vi "ni5660 Read FFT Spectrum.vi"(0 "receiver info in":T2, 9 "correction factor":T1[](array[typedef]) {"spectrum correction"."correction factors" format="%.2f"; "spectrum correction"."df" format="%.2f"; "spectrum correction"."f0" format="%.2f"}, 11 "error in (no error)":errorcluster) -> (4 "receiver info out":T2, 6 "FFT spectrum (Vrms)":cluster{"f0":dbl, "df":dbl, "spectrum":cdb[]} {"spectrum" format="%.2f"; "df" format="%.2f"; "f0" format="%.2f"}, 8 "spectral info out":T3={"spectrum type"=enum."Power [Magnitude^2]", "linear/dB"=enum."linear", "window"=0, "window size"=1024, "FFT size"=1024} {"window" items=["None ", "Hanning", "Hamming", "Blackman-Harris", "Exact Blackman", "Blackman", "Flat Top", "4 Term B-Harris ", "7 Term B-Harris", "Low Sidelobe"]}, 15 "error out":errorcluster)   [LabVIEW 2011]
doc: "This VI computes the FFT spectrum that corresponds to the spectral settings specified in the ni5660 Configure for Spectrum VI. The VI returns a cluster that contains the FFT spectrum in Vrms, starting at frequency <B>f0</B> and frequency interval <B>df</B>. Wire the <B>FFT spectrum</B> output to averaging and/or measurement VIs in the Spectral Measurements Toolkit."
uses:
  <vilib>/measure/masml.llb/ma_sml_Spectral Info.ctl
  <vilib>/addons/Modulation/niScope/controls/mod_Modulation Settings.ctl
  <vilib>/addons/Spectral Measurements Toolset/LVSupport/SMT niScope Utilities/smt_correction.ctl
  <vilib>/addons/Spectral Measurements Toolset/LVSupport/SMT niScope Utilities/smt_Apply Correction(FFT).vi
  <vilib>/addons/Spectral Measurements Toolset/SMT Zoom FFT for niScope.vi
  <vilib>/measure/NI_MAPro.lvlib
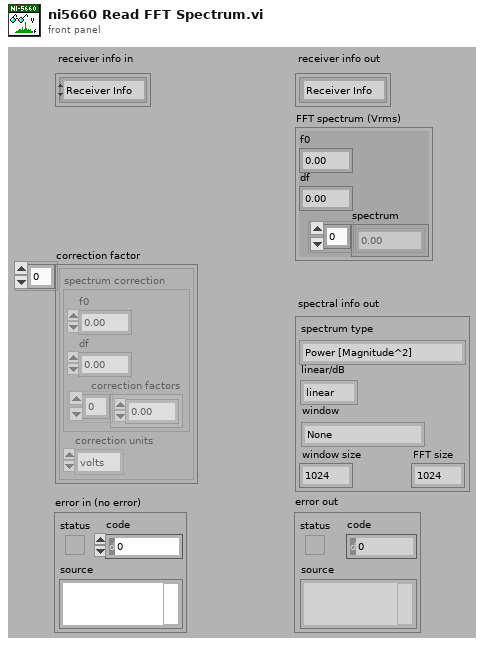
[diagram p1: front panel]
types:
  T1 = typedef "smt_correction.ctl" = cluster{"spectrum correction":cluster{"f0":dbl, "df":dbl, "correction factors":dbl[]}, "correction units":enum16{"volts", "watts", "dB"}}
  T2 = typedef "mod_Modulation Settings.ctl" = cluster{enum16{"Receiver Info"}, variant}
  T3 = typedef "NI_MAPro.lvlib/ma_sml_Spectral Info.ctl" = cluster{"spectrum type":enum16{"FFT Spectrum [complex]", "Amplitude [Magnitude]", "Power [Magnitude^2]", "Cross Spectrum [complex]", "Frequency Response [Complex]"}, "linear/dB":enum16{"linear", "dB"}, "window":u16, "window size":i32, "FFT size":i32}
  T4 = enum16{"V", "V^2", "W", "dBm", "dBW", "dBV", "dBmV", "dBuV"}
  T5 = typedef "mod_Readable Attributes Cluster.ctl" = cluster{"carrier":cluster{"frequency":dbl}, "receiver":cluster{"handles":cluster{"niTuner taskID":i32, "niScope handle":refnum<k15>}, "RFSA":cluster{"reference level":i32, "RF attenuation":i32}, "data format":enum16{"real", "complex modulated (array)", "complex modulated (interleaved)"}, "auto suppress SW IQ":enum16{"off", "on"}, "IQ sample rate":dbl, "bandwidth":dbl}}
  T6 = cluster{"multispan?":bool, "segment size":dbl, "number of segments":i32, "frequency shifts":dbl[], "fc adjustment":dbl, "df":dbl, "start frequency (Hz)":dbl, "stop frequency (Hz)":dbl}
  T7 = typedef "NI_MAPro.lvlib/ma_sml_ND Zoom FFT Settings.ctl" = cluster{"zoom settings":cluster{"center frequency":dbl, "zoom":i32, "trim":dbl}, "FFT settings":cluster{"window":u16, "FFT size":i32}}
  T8 = cluster{"zoom FFT settings":T7, "frequency shift":dbl, "data format":enum16{"real", "complex modulated (array)", "complex modulated (interleaved)"}}
  T9 = cluster{"relativeInitialX":dbl, "xIncrement":dbl, "wfm":dbl[]}[]
  T10 = typedef "NI_MAPro.lvlib/ma_sml_Spectrum Cluster (complex).ctl" = cluster{"f0":dbl, "df":dbl, "spectrum":cdb[]}
  T11 = cluster{"spectrum type":enum16{"FFT Spectrum [complex]", "Amplitude [Magnitude]", "Power [Magnitude^2]", "Cross Spectrum [complex]", "Frequency Response [Complex]"}, "linear/dB":enum16{"linear", "dB"}, "window":enum16{"None ", "Hanning", "Hamming", "Blackman-Harris", "Exact Blackman", "Blackman", "Flat Top", "4 Term B-Harris ", "7 Term B-Harris", "Low Sidelobe"}, "window size":i32, "FFT size":i32}
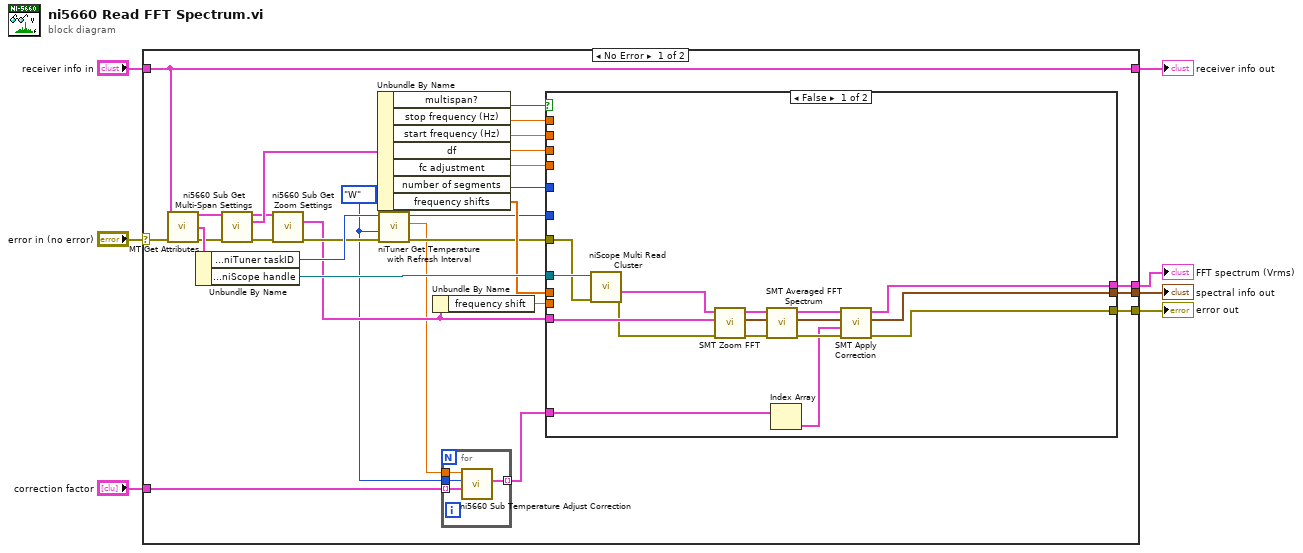
[diagram p0: block diagram]
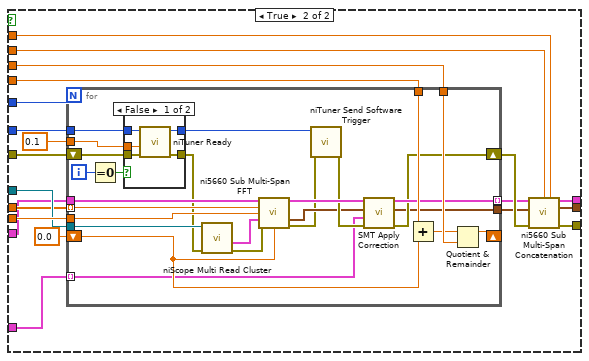
[diagram p2: hidden frame]
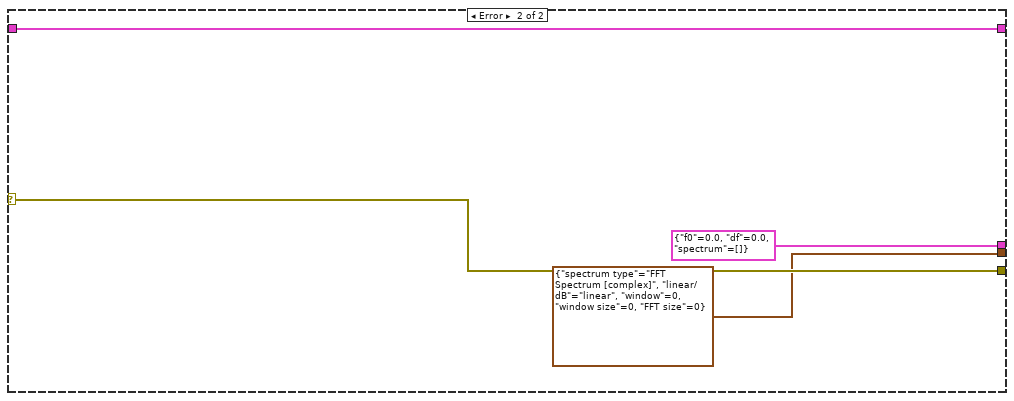
[diagram p4: hidden frame]
diagram:
  n1 = case shown="No Error" "error in (no error)" {
    selector: "error in (no error)" -> [w30 w113]
    tunnel: [w36 w113] -> w7
    tunnel: "correction factor" -> [w35 _]
    tunnel: [w8 cluster{"f0":dbl, "df":dbl, "spectrum":cdb[]} {"f0"=0.0, "df"=0.0, "spectrum"=[]} ("corrected FFT spectrum")] -> w1
    tunnel: [w34 T3 {"spectrum type"=enum."FFT Spectrum [complex]", "linear/dB"=enum."linear", "window"=0, "window size"=0, "FFT size"=0} ("spectral info out")] -> w5
    tunnel: "receiver info in" -> [w29 w112]
    tunnel: [w29 w112] -> w3
    frame No Error {
      w10 = T4."W" ("correction units")
      n2 = call <vilib>:"MT Get Attributes.vi"("receiver info in"=w29, "error in (no error)"=w30) -> ("receiver info out"=w28:T2, "attributes"=w33:T5, "error out"=w27:errorcluster)  [unwired: 11 in]
      n3 = Unbundle By Name(w33) -> ("receiver.handles.niTuner taskID"=w31:i32, "receiver.handles.niScope handle"=w32:refnum<k15>)
      n4 = call <instrlib>:"ni5660 Sub Get Multi-Span Settings.vi"("receiver info in"=w28, "error in (no error)"=w27) -> ("receiver info out"=w24:T2, "multispan settings"=w26:T6, "error out"=w25:errorcluster)  [unwired: 10 in, 1 out]
      n5 = call <instrlib>:"ni5660 Sub Get Zoom Settings.vi"("receiver info in"=w24, "error in (no error)"=w25) -> ("zoom settings"=w22:T8, "error out"=w23:errorcluster)  [unwired: 10 in, 2 out]
      n6 = Unbundle By Name(w26) -> ("multispan?"=w14:bool, "stop frequency (Hz)"=w15:dbl, "start frequency (Hz)"=w20:dbl, "df"=w19:dbl, "fc adjustment"=w18:dbl, "number of segments"=w9:i32, "frequency shifts"=w17:dbl[])
      n7 = call <instrlib>:"niTuner Get Temperature with Refresh Interval.vi"("error in"=w23, "correction units"=w10, "taskID in"=w31) -> ("error out"=w12:errorcluster, "correction factor"=w11:dbl, "taskID out"=w13:i32)  [unwired: 5 in, 1 out]
      n8 = Unbundle By Name(w22) -> ("frequency shift"=w21:dbl)
      n9 = for {
        tunnel: [w40] -> w16 mode=indexing
        tunnel: w35 -> [w39] mode=indexing
        tunnel: w11 -> [w38]
        tunnel: w10 -> [w37]
        n10 = call <instrlib>:"ni5660 Sub Temperature Adjust Correction.vi"("correction"=w39, "temperature correction units"=w37, "temperature correction factor"=w38) -> ("temperature adjusted correction"=w40:T1)  [unwired: 8 in]
      }
      n11 = case shown="False" w14 {
        tunnel: w21 -> [_ w76]
        tunnel: w32 -> [w56 w71]
        tunnel: w20 -> [_ w70]
        tunnel: w19 -> [_ w69]
        tunnel: w18 -> [_ w68]
        tunnel: w17 -> [_ w67]
        tunnel: w16 -> [w54 w66]
        tunnel: [w52 w65] -> w36
        tunnel: w15 -> [_ w64]
        tunnel: [w47 w60] -> w8
        tunnel: [w53 w63] -> w34
        tunnel: w12 -> [w41 w59]
        tunnel: w13 -> [_ w58]
        tunnel: w22 -> [w50 w62]
        tunnel: w9 -> [_ w61]
        frame False {
          n12 = call <instrlib>:"niScope Multi Read Cluster.vi"("error in"=w41, "instrument handle"=w56) -> ("error out"=w46:errorcluster, "waveform"=w44:T9)  [unwired: 6 in, 2 out]
          n13 = call-poly <vilib>:"SMT Zoom FFT.vi"("error in (no error)"=w46, "SMT zoom settings"=w50, "waveforms"=w44) -> ("error out"=w45:errorcluster, "spectral info"=w42:T3, "FFT spectrum (Vrms)"=w43:T10)  [unwired: 6 in]
          n14 = call <vilib>:"SMT Averaged FFT Spectrum.vi"("error in (no error)"=w45, "spectral info in"=w42, "FFT spectrum"=w43) -> ("error out"=w55:errorcluster, "spectral info out"=w49:T11, "averaged FFT spectrum"=w48:cluster{"f0":dbl, "df":dbl, "spectrum":cdb[]})  [unwired: 4 in, 2 out]
          n15 = Index Array(array=w54) -> (element=w51:T1)  [unwired: 1 in]
          n16 = call-poly <vilib>:"SMT Apply Correction.vi"("error in (no error)"=w55, "correction"=w51, "spectral info in"=w49, "FFT spectrum"=w48) -> ("error out"=w52:errorcluster, "spectral info out"=w53:T3, "corrected FFT spectrum"=w47:cluster{"f0":dbl, "df":dbl, "spectrum":cdb[]})  [unwired: 5 in]
        }
        frame True {
          n17 = for {
            N: w61 -> [_]
            tunnel: w71 -> [w96]
            tunnel: [w87] -> w73
            tunnel: w67 -> [w94] mode=indexing
            shift-right: [w97] -> _
            shift-left: 0.0 ("timeout") -> [w92]
            tunnel: w68 -> [w101]
            tunnel: w69 -> [w102]
            shift-right: [w88] -> w75
            shift-left: w59 -> [w98]
            tunnel: w62 -> [w95]
            tunnel: w76 -> [w93]
            tunnel: w66 -> [w86] mode=indexing
            tunnel: [w89] -> w72 mode=indexing
            tunnel: w58 -> [w81]
            tunnel: 0.1 ("timeout") -> [w80]
            i -> [w77]
            n18 = Equal To 0?(x=w77) -> (x = 0?=w78:bool)
            n19 = case shown="False" w78 {
              tunnel: [w107 w108] -> w99
              tunnel: w98 -> [w106 w109]
              tunnel: w81 -> [w105 w108]
              tunnel: w80 -> [w104 _]
              tunnel: [w103 w109] -> w79
              frame False {
                n20 = call <instrlib>:"niTuner Ready.vi"("error in"=w106, "timeout"=w104, "taskID in"=w105) -> ("error out"=w103:errorcluster, "taskID out"=w107:i32)  [unwired: 6 in, 1 out]
              }
              frame True {
              }
            }
            n21 = call <instrlib>:"niScope Multi Read Cluster.vi"("error in"=w79, "instrument handle"=w96) -> ("error out"=w84:errorcluster, "waveform"=w83:T9)  [unwired: 6 in, 2 out]
            n22 = call <instrlib>:"ni5660 Sub Multi-Span FFT.vi"("SMT zoom settings"=w95, "Tuner Frequency Shift"=w94, "DDC Frequency Shift"=w93, "waveform"=w83, "error in (no error)"=w84, "fc adjust"=w92) -> ("averaged FFT spectrum"=w91:cluster{"f0":dbl, "df":dbl, "spectrum":cdb[]}, "spectral info in"=w85:T11, "error out"=w82:errorcluster)  [unwired: 5 in, 2 out]
            n23 = call <instrlib>:"niTuner Send Software Trigger.vi"("error in"=w82, "taskID in"=w99) -> ("error out"=w90:errorcluster)  [unwired: 8 in, 1 out]
            n24 = call-poly <vilib>:"SMT Apply Correction.vi"("error in (no error)"=w90, "correction"=w86, "spectral info in"=w85, "FFT spectrum"=w91) -> ("error out"=w88:errorcluster, "spectral info out"=w87:T3, "corrected FFT spectrum"=w89:cluster{"f0":dbl, "df":dbl, "spectrum":cdb[]})  [unwired: 5 in]
            n25 = Add(x=w101, y=w92) -> (x+y=w100:dbl)
            n26 = Quotient & Remainder(x=w100, y=w102) -> (x-y*floor(x/y)=w97:dbl)  [unwired: 1 out]
          }
          n27 = call <instrlib>:"ni5660 Sub Multi-Span Concatenation.vi"("FFT spectrum array"=w72, "Fstart"=w70, "Fstop"=w64, "spectral info in"=w73, "error in (no error)"=w75) -> ("concatenated FFT spectrum"=w60:cluster{"f0":dbl, "df":dbl, "spectrum":cdb[]}, "spectral info out"=w63:T3, "error out"=w65:errorcluster)  [unwired: 7 in, 1 out]
        }
      }
    }
    frame Error {
    }
  }
  "error out" <- w7
  "spectral info out" <- w5
  "receiver info out" <- w3
  "FFT spectrum (Vrms)" <- w1
